vi "Controller.vi"(5 "PID gain schedule":T1(array[cluster])=[{"PID gains"={"proportional gain (Kc)"=1.0, "integral time (Ti, min)"=0.01, "derivative time (Td, min)"=0.0}, "max value"=100.0}] {"max value" format="%.2f"; "PID gains"."derivative time (Td, min)" format="%.6f"; "PID gains"."integral time (Ti, min)" format="%.6f"; "PID gains"."proportional gain (Kc)" format="%.6f"}, 6 "error in (no error)":errorcluster, 7 "setpoint profile":cluster{"time (s)":dbl, "setpoint":dbl}[](array[cluster]), 9 "Process_REF":string="Temperature") -> (0 "error out":errorcluster)   [LabVIEW 2018]
uses:
  <vilib>/addons/control/pid/pid.llb/PID Gain Schedule (DBL).vi
  <vilib>/addons/control/pid/pid.llb/PID Advanced (DBL).vi
  <vilib>/addons/control/pid/NI_PID_pid.lvlib
panel:
  in  "Reinitialize Profile":bool
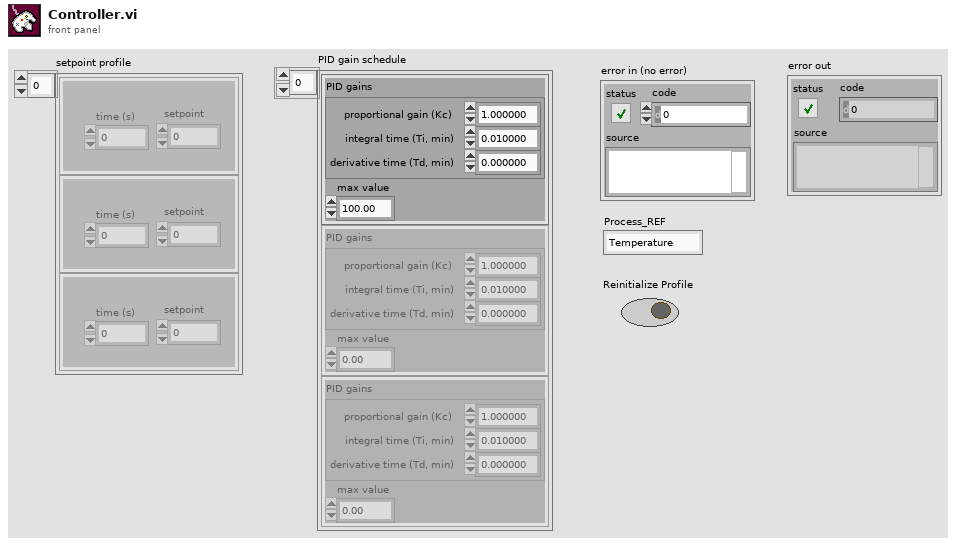
[diagram p1: front panel]
types:
  T1 = cluster{"PID gains":cluster{"proportional gain (Kc)":dbl, "integral time (Ti, min)":dbl, "derivative time (Td, min)":dbl}, "max value":dbl}[]
  T2 = cluster{"proportional gain (Kc)":dbl, "integral time (Ti, min)":dbl, "derivative time (Td, min)":dbl}
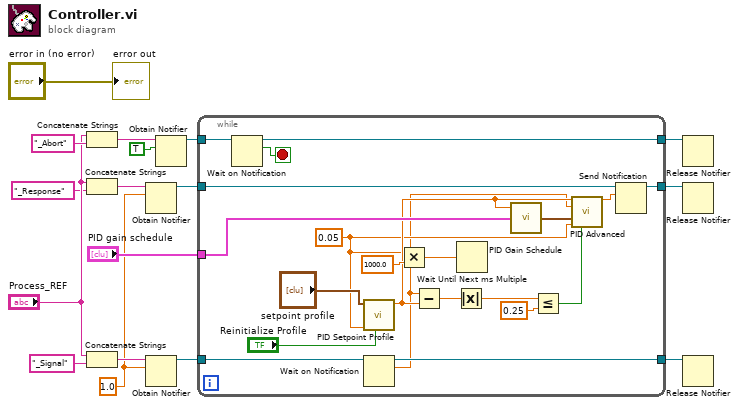
[diagram p0: block diagram]
diagram:
  w3 = 1.0
  n1 = Concatenate Strings("Process_REF", "_Abort") -> (w8:string)
  n2 = Concatenate Strings("Process_REF", "_Response") -> (w6:string)
  n3 = Concatenate Strings("Process_REF", "_Signal") -> (w4:string)
  n4 = Obtain Notifier(name (unnamed)=w6, notification data type=w3) -> (notifier out=w5:refnum<notifier>)  [unwired: 2 in, 2 out]
  n5 = Obtain Notifier(name (unnamed)=w4, notification data type=w3) -> (notifier out=w2:refnum<notifier>)  [unwired: 2 in, 2 out]
  n6 = Obtain Notifier(name (unnamed)=w8, notification data type=TRUE) -> (notifier out=w7:refnum<notifier>)  [unwired: 2 in, 2 out]
  n7 = while {
    tunnel: "PID gain schedule" -> [w37]
    tunnel: w2 -> [w18]
    tunnel: w7 -> [w22]
    tunnel: [w20] -> w10
    tunnel: [w23] -> w1
    tunnel: w5 -> [w24]
    tunnel: [w25] -> w11
    stop <- w21 stop-if-true
    w27 = 0.05
    n8 = Wait on Notification(notifier=w22) -> (notifier out=w23:refnum<notifier>, notification=w21:bool)  [unwired: 3 in, 2 out]
    n9 = call <vilib>:"PID Setpoint Profile.vi"("reinitialize? (F)"="Reinitialize Profile", "dt (s)"=w27, "setpoint profile"="setpoint profile") -> ("setpoint"=w33:dbl)  [unwired: 3 in, 3 out]
    n10 = Wait on Notification(notifier=w18) -> (notifier out=w20:refnum<notifier>, notification=w19:dbl)  [unwired: 3 in, 2 out]
    n11 = Multiply(x=w27, y=1000.0) -> (x*y=w35:dbl)
    n12 = Subtract(x=w19, y=w33) -> (x-y=w32:dbl)
    n13 = Absolute Value(x=w32) -> (abs(x)=w31:dbl)
    n14 = Wait Until Next ms Multiple(millisecond multiple=w35) -> ()  [unwired: 1 out]
    n15 = call-poly <vilib>:"PID Gain Schedule.vi"("PID gain schedule"=w37, "gain scheduling value"=w33) -> ("PID gains out"=w38:T2)  [unwired: 2 in, 1 out]
    n16 = Less Or Equal?(x=w31, y=0.25) -> (x <= y?=w29:bool)
    n17 = call-poly <vilib>:"PID Advanced.vi"("setpoint"=w33, "process variable"=w19, "PID gains"=w38, "dt (s)"=w27, "reinitialize? (F)"=w29) -> ("output"=w26:dbl)  [unwired: 9 in, 1 out]
    n18 = Send Notification(notification=w26, notifier=w24) -> (notifier out=w25:refnum<notifier>)  [unwired: 1 in, 1 out]
  }
  n19 = Release Notifier(notifier=w1) -> ()  [unwired: 2 in, 3 out]
  n20 = Release Notifier(notifier=w11) -> ()  [unwired: 2 in, 3 out]
  n21 = Release Notifier(notifier=w10) -> ()  [unwired: 2 in, 3 out]
  "error out" <- "error in (no error)"
